vi "ParseMeta.vi"(0 "Path":path, 7 "Instrument":u16(ring) items=["Unknown", "Phillips SEM IRC", "JEOL 7000F EML_MFC", "MXRD MFC", "JEOL_EPMA"], 12 "Spot_info_in":T1) -> (4 "X-stage (um)":dbl, 6 "Y-stage (um)":dbl, 8 "Z-stage (um)":dbl, 10 "R-stage (deg)":dbl, 14 "Spot_info_out":T1, 15 "StageTilt":dbl)   [LabVIEW 2011]
doc: "Parses some basic information for files that contain meta information about data for various insturments. Current supports Phillips TIFF, Bruker XRD uxd files, and EMSA files as produced by Oxford INCA software for the JEOL 7000"
uses:
  cm2nm_coordinate_information_v2.ctl
panel:
  out "submatch 2":string
  out "Picture":picture
  out "error out":errorcluster
  out "match substring":string
  out "data":string
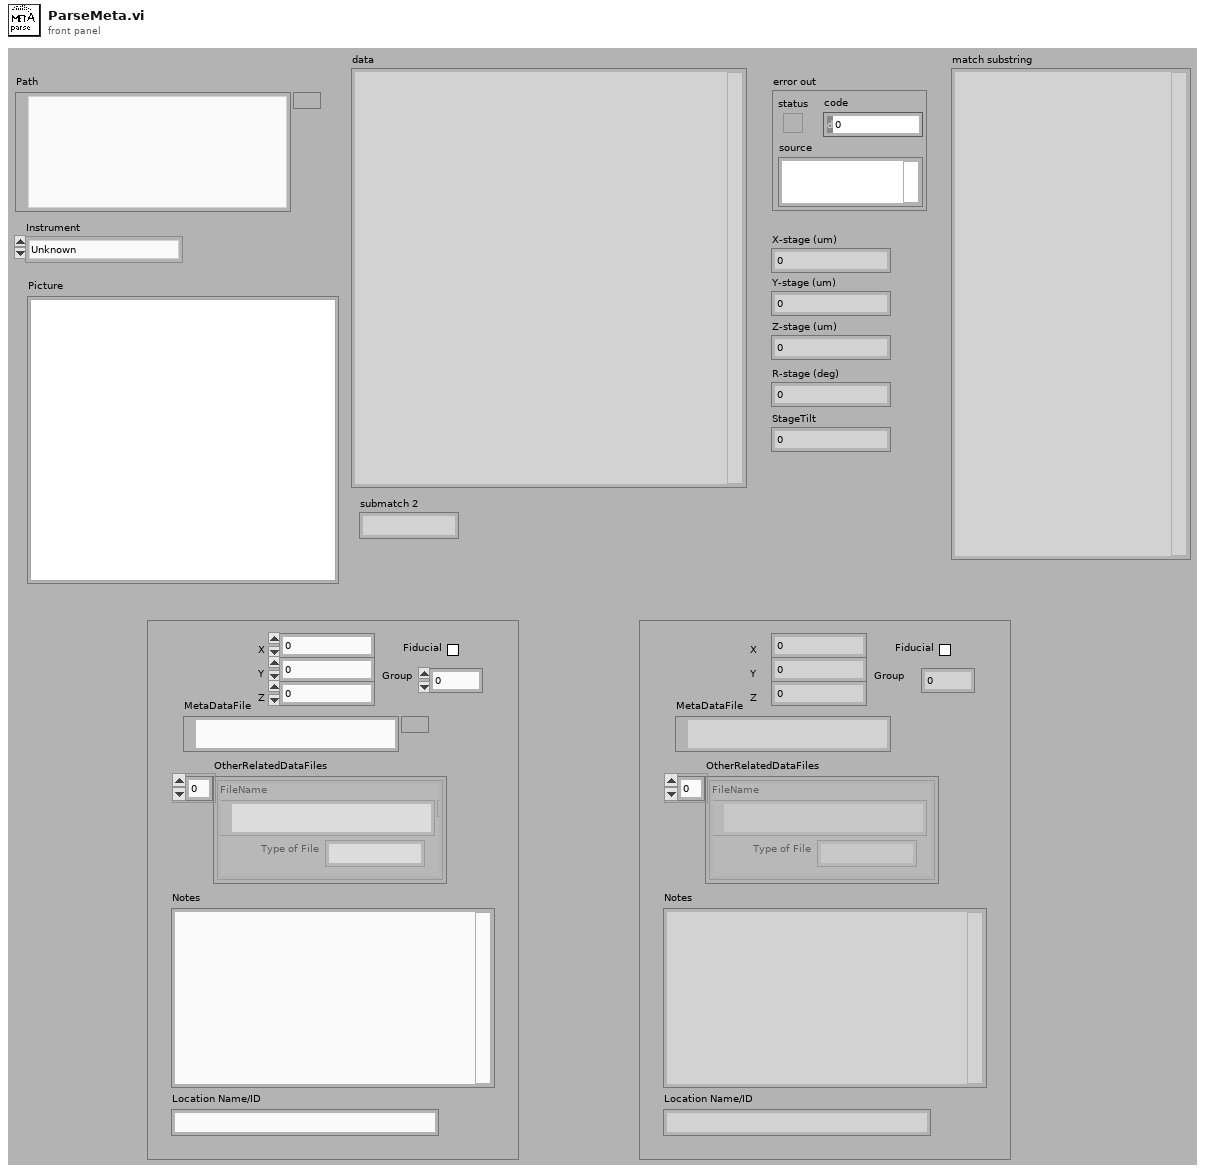
[diagram p1: front panel]
types:
  T1 = typedef "cm2nm_coordinate_information_v2.ctl" = cluster{"MetaDataFile":path, "X":dbl, "Y":dbl, "Z":dbl, "Group":i32, "Rotation":dbl[unit], "Fiducial":bool, "Magnification":dbl, "Working_Distance":dbl, "Notes":string, "Location Name/ID":string, "OtherRelatedDataFiles":cluster{"Type of File":string, "FileName":path}[], "Available":bool}
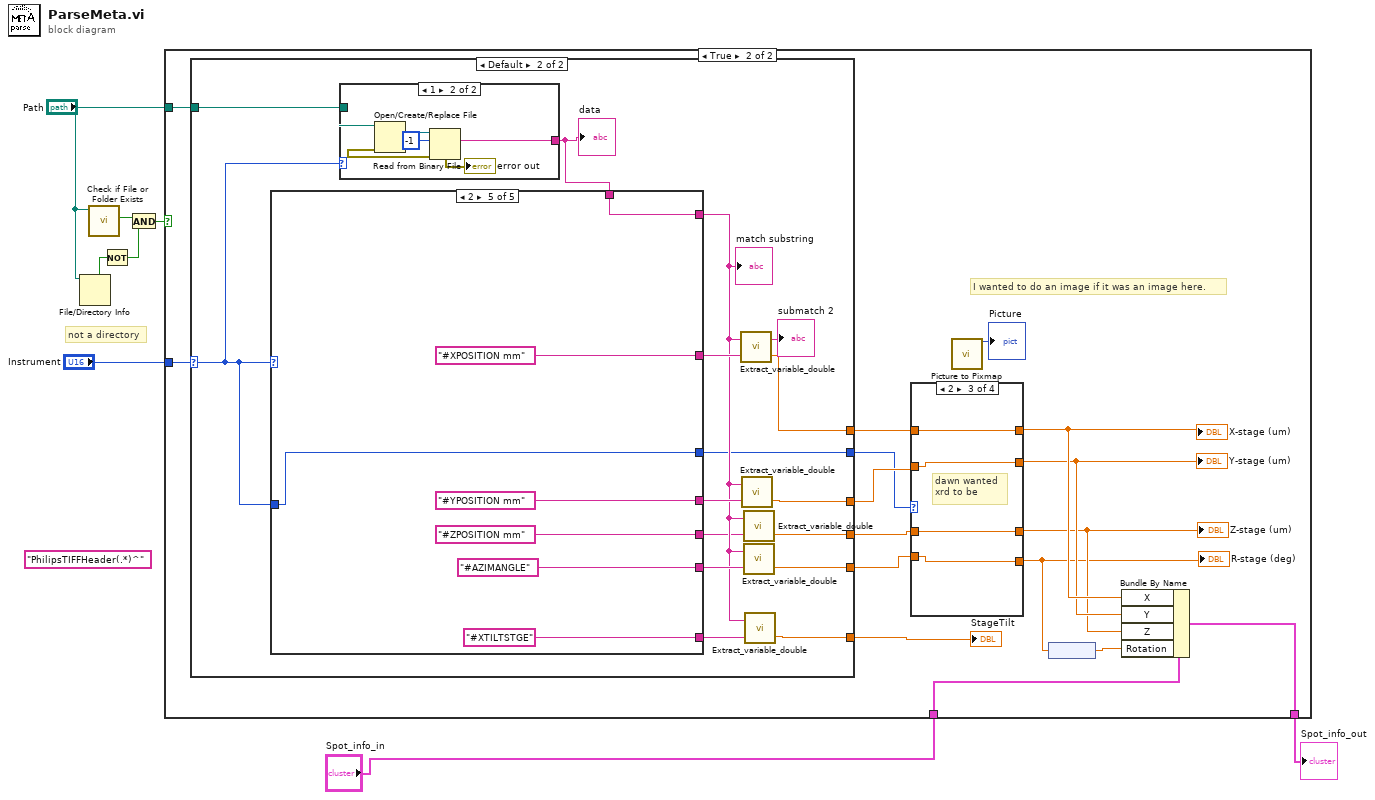
[diagram p0: block diagram]
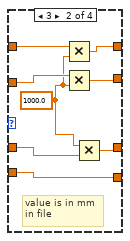
[diagram p4: hidden frame]
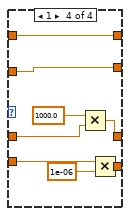
[diagram p5: hidden frame]
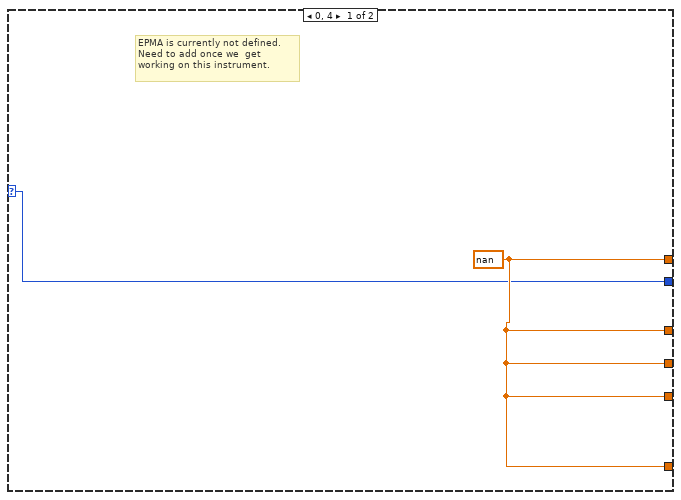
[diagram p6: hidden frame]
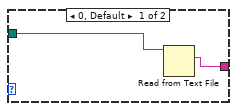
[diagram p7: hidden frame]
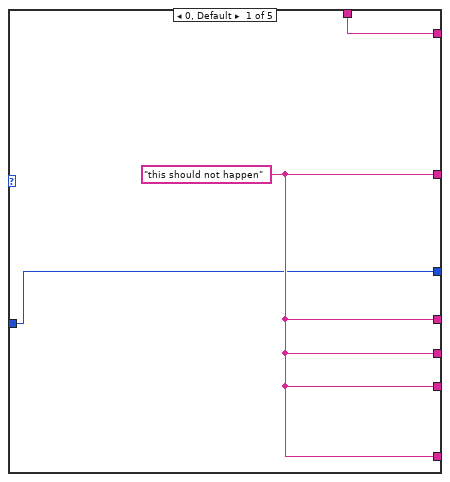
[diagram p8: hidden frame]
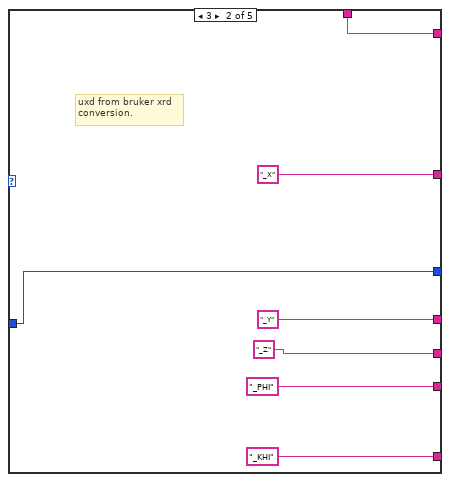
[diagram p9: hidden frame]
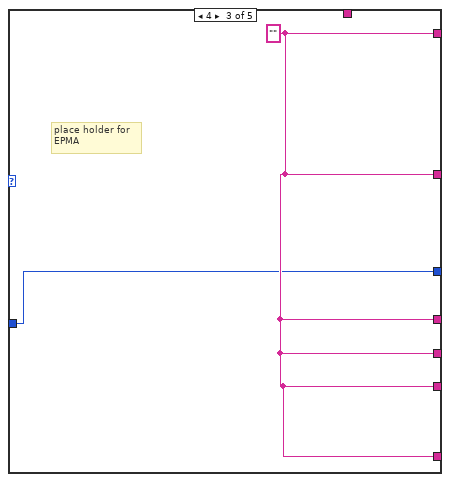
[diagram p10: hidden frame]
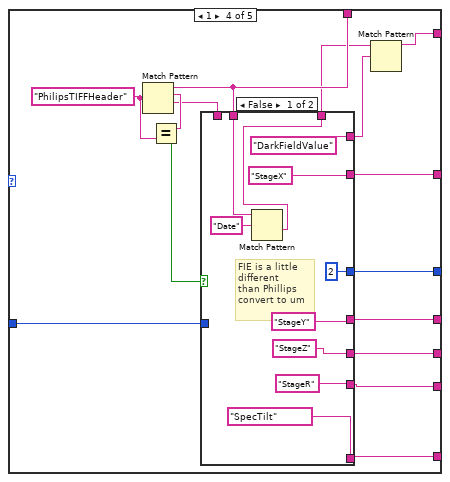
[diagram p11: hidden frame]
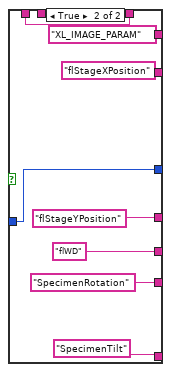
[diagram p12: hidden frame]
diagram:
  (unwired) "PhilipsTIFFHeader(.*)^" ("regular expression")
  # "not a directory"
  n1 = File/Directory Info(path="Path") -> (directory=w1:bool)  [unwired: 1 in, 6 out]
  n2 = call <vilib>:"Check if File or Folder Exists.vi"("path"="Path") -> ("file or folder exists?"=w6:bool)  [unwired: 1 in, 9 out]
  n3 = Not(x=w1) -> (.not. x?=w7:bool)
  n4 = And(x=w6, y=w7) -> (x .and. y?=w5:bool)
  n5 = case shown="True" w5 {
    tunnel: "Instrument" -> [_ w19]
    tunnel: "Path" -> [_ w17]
    tunnel: "Spot_info_in" -> [w9 w16]
    tunnel: [w9 w15] -> w3
    frame False {
    }
    frame True {
      # "I wanted to do an image if it was an image here."
      n6 = case shown="Default" w19 {
        selector: w19 -> [w50 w55]
        tunnel: [w51 w67] -> w21
        tunnel: [w51 w66] -> w24
        tunnel: [w51 w65] -> w23
        tunnel: [w51 w64] -> w20
        tunnel: [w51 w56] -> w22
        tunnel: [w50 w54] -> w18
        tunnel: w17 -> [_ w52]
        frame 0, 4 {
          w51 = nan ("Output")
          # "EPMA is currently not defined.\nNeed to add once we  get \nworking on this instrument."
        }
        frame Default {
          n7 = case shown="1" w55 {
            tunnel: [w68 w74] -> w53
            tunnel: w52 -> [w69 w71]
            frame 0, Default {
              n8 = Read from Text File(file (use dialog)=w69) -> (text=w68:string)  [unwired: 1 in, 5 out]
            }
            frame 1 {
              n9 = Open/Create/Replace File(file path (use dialog)=w71) -> (refnum out=w75:refnum<file>, error out=w72:errorcluster)  [unwired: 1 in, 5 out]
              n10 = Read from Binary File(8:w72, 10:-1 ("count (1)"), 11:w75) -> (0:→"error out":errorcluster, 2:w74:string)  [unwired: 5 out]
            }
          }
          "data" <- w53
          n11 = case shown="2" w55 {
            tunnel: w53 -> [w78 w85 _ w91 w127]
            tunnel: [w77 "_X" ("string") w87 w101 "#XPOSITION mm" ("string")] -> w63
            tunnel: [w77 "_Y" ("string") w87 w100 "#YPOSITION mm" ("string")] -> w61
            tunnel: [w77 "_PHI" ("string") w87 w99 "#AZIMANGLE" ("string")] -> w60
            tunnel: [w77 "_KHI" ("string") w87 w98 "#XTILTSTGE" ("string")] -> w59
            tunnel: [w78 w85 w87 w97 w127] -> w58
            tunnel: [w77 "_Z" ("string") w87 w96 "#ZPOSITION mm" ("string")] -> w57
            tunnel: w55 -> [w76 w79 w86 w89 w121]
            tunnel: [w76 w79 w86 w88 w121] -> w54
            frame 0, Default {
              w77 = "this should not happen" ("string")
            }
            frame 3 {
              # "uxd from bruker xrd\nconversion."
            }
            frame 4 {
              w87 = ""
              # "place holder for \nEPMA"
            }
            frame 1 {
              w94 = "PhilipsTIFFHeader" ("regular expression")
              n12 = Match Pattern(string=w91, regular expression=w94) -> (match substring=w95:string, after substring=w92:string)  [unwired: 3 out]
              n13 = Equal?(x=w95, y=w94) -> (x = y?=w93:bool)
              n14 = case shown="False" w93 {
                tunnel: ["DarkFieldValue" "XL_IMAGE_PARAM" ("regular expression")] -> w102
                tunnel: ["StageX" "flStageXPosition" ("string")] -> w101
                tunnel: ["StageY" "flStageYPosition" ("string")] -> w100
                tunnel: ["StageR" "SpecimenRotation" ("string")] -> w99
                tunnel: ["SpecTilt" ("string") "SpecimenTilt" ("string")] -> w98
                tunnel: ["StageZ" "flWD" ("string")] -> w96
                tunnel: w92 -> [_ w114]
                tunnel: w91 -> [w106 _]
                tunnel: [w104 w114] -> w90
                tunnel: w89 -> [_ w113]
                tunnel: [u16 2 ("Instrument") w113] -> w88
                frame False {
                  # "FIE is a little\ndifferent\nthan Phillips\nconvert to um"
                  n15 = Match Pattern(string=w106, regular expression="Date") -> (after substring=w104:string)  [unwired: 4 out]
                }
                frame True {
                }
              }
              n16 = Match Pattern(string=w90, regular expression=w102) -> (before substring=w97:string)  [unwired: 4 out]
            }
            frame 2 {
            }
          }
          "match substring" <- w58
          n17 = call "Extract_variable_double.vi"("key"=w63, "InputString"=w58) -> ("Output"=w67:dbl, "outstring"=→"submatch 2":string)
          n18 = call "Extract_variable_double.vi"("key"=w61, "InputString"=w58) -> ("Output"=w64:dbl)  [unwired: 1 out]
          n19 = call "Extract_variable_double.vi"("key"=w57, "InputString"=w58) -> ("Output"=w56:dbl)  [unwired: 1 out]
          n20 = call "Extract_variable_double.vi"("key"=w60, "InputString"=w58) -> ("Output"=w66:dbl)  [unwired: 1 out]
          n21 = call "Extract_variable_double.vi"("key"=w59, "InputString"=w58) -> ("Output"=w65:dbl)  [unwired: 1 out]
        }
      }
      "StageTilt" <- w23
      n22 = case shown="2" w18 {
        tunnel: w24 -> [w29 w32 w38 w49]
        tunnel: [w29 w32 w38 w48] -> w11
        tunnel: w22 -> [w28 w31 w39 w46]
        tunnel: [w28 w33 w39 w44] -> w12
        tunnel: w21 -> [w27 w37 w41 w43]
        tunnel: [w27 w36 w41 w43] -> w14
        tunnel: w20 -> [w26 w34 w40 w42]
        tunnel: [w26 w35 w40 w42] -> w13
        frame 0, Default {
        }
        frame 3 {
          w30 = 1000.0 ("y")
          # "value is in mm\nin file"
          n23 = Multiply(x=w37, y=w30) -> (x*y=w36:dbl)
          n24 = Multiply(x=w34, y=w30) -> (x*y=w35:dbl)
          n25 = Multiply(x=w30, y=w31) -> (x*y=w33:dbl)
        }
        frame 2 {
          # "dawn wanted\nxrd to be"
        }
        frame 1 {
          n26 = Multiply(x=1000.0, y=w46) -> (x*y=w44:dbl)
          n27 = Multiply(x=w49, y=1e-06) -> (x*y=w48:dbl)
        }
      }
      "X-stage (um)" <- w14
      "R-stage (deg)" <- w11
      "Y-stage (um)" <- w13
      "Z-stage (um)" <- w12
      n28 = call <vilib>:"Picture to Pixmap.vi"() -> ("new picture"=→"Picture":picture)  [unwired: 4 in, 7 out]
      n29 = node(w11) -> (w10:dbl[unit])
      n30 = Bundle By Name(cluster=w16, "X"=w14, "Y"=w13, "Z"=w12, "Rotation"=w10) -> (w15:T1)
    }
  }
  "Spot_info_out" <- w3
